vi "(auto) Analyze pattern.vi"(8 "Pattern classes":i32[](array[numeric]), 9 "Image In":T1, 10 "ROI Descriptor (Image Mask 1)":T2, 11 "pattern number":i32=1) -> (0 "output array":i32[](array[numeric]), 1 "Image Out":T1, 2 "Pattern":i32)   [LabVIEW 2017]
uses:
  <vilib>/vision/Image Controls.llb/IMAQ Image.ctl
panel:
  in  "millisecond timer value":u32
  # "out"
  # "in"
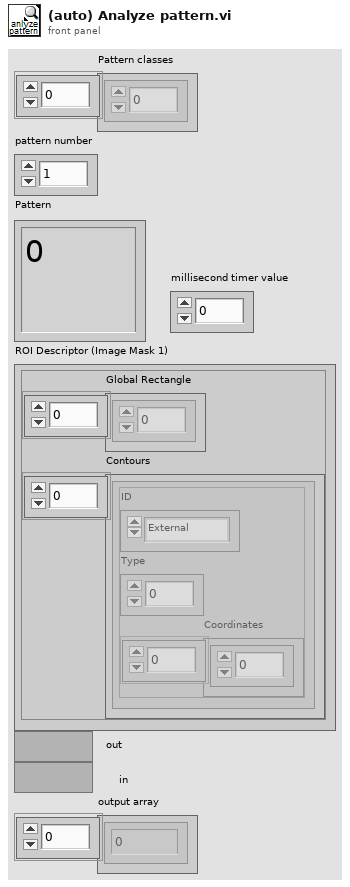
[diagram p1: front panel]
types:
  T1 = typedef "IMAQ Image.ctl" = refnum<image>
  T2 = cluster{"Global Rectangle":i32[], "Contours":cluster{"ID":enum32{"External", "Internal"}, "Type":u32, "Coordinates":i32[]}[]}
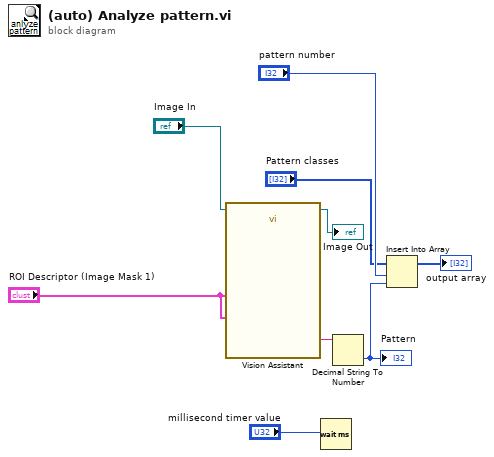
[diagram p0: block diagram]
diagram:
  n1 = call "Vision Assistant"("Image In"="Image In", "ROI Descriptor (Image Mask 1)"="ROI Descriptor (Image Mask 1)", "ROI Descriptor (Particle Classification 1)"="ROI Descriptor (Image Mask 1)") -> ("Image Out"=→"Image Out":T1, "Class (Particle Classification 1)"=w8:string)  [unwired: 22 in, 1 out]
  n2 = Wait (ms)(milliseconds to wait="millisecond timer value") -> ()  [unwired: 1 out]
  n3 = Decimal String To Number(string=w8) -> (number=w9:i32)  [unwired: 2 in, 1 out]
  "Pattern" <- w9
  n4 = Insert Into Array(array="Pattern classes", index="pattern number", new element=w9) -> (→"output array":i32[])
